vi "prepAO_imgtest.vi"() -> (0 "size(s)":i32[](array[numeric]))   [LabVIEW 2013]
uses:
  <vilib>/DAQmx/write.llb/DAQmx Write (Analog 2D DBL NChan NSamp).vi
  <vilib>/DAQmx/write.llb/DAQmx Write (Analog 1D DBL 1Chan NSamp).vi
  <vilib>/DAQmx/create/channels.llb/DAQmx Create Channel (AO-Voltage-Basic).vi
  <vilib>/DAQmx/configure/timing.llb/DAQmx Timing (Sample Clock).vi
  <vilib>/DAQmx/miscellaneous.llb/DAQmx Fill In Error Info.vi
  <resource>/objmgr/daqmx.rc
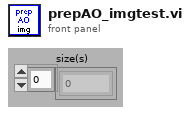
[diagram p1: front panel]
types:
  T1 = cluster{"Min Voltage sq (mV)":dbl, "Max voltage sq (mV)":dbl, "Duty cycle sq(%)":dbl, "Voltage freq. sq(Hz)":dbl, "# cycles sq":u32, "meastype":enum16{"sealtest hekcells", "sealtest neurons", "Manual", "from file"}, "sample rate":dbl, "amp":dbl, "sample mode":i32, "refreshbuffer":i32, "timeout":sgl, "patch":bool, "laserAO":bool, "shutter":bool, "488":bool, "532":bool, "640":bool, "Min Voltage tri (mV)":dbl, "Max voltage tri (mV)":dbl, "Voltage freq. tri(Hz)":dbl, "# cycles tri":u32, "Voltage step ":bool, "Voltage triangle":bool, "file":bool, "refreshrate":dbl, "sAOXY":dbl, "avpp":i32}
  T2 = cluster{"CH1 AI":tag, "CH1 CI":tag, "CH2 AI":tag, "CH2 CI":tag, "AI X":tag, "AI Y":tag, "AO X-Y":tag, "CH1ST":bool, "CH2ST":bool, "Sigcase":i16, "StageS":i32, "StageL":i32, "data dir":path, "Vp":tag, "Ip":tag, "AO CWlaser":tag, "AO VtoP":tag, "shutter":tag, "LT marker":tag, "488":tag, "532":tag, "640":tag}
  T3 = cluster{"Xpixels":i32, "Vx-min ref":dbl, "Vx-max ref":dbl, "P":dbl, "Ypixels":i32, "Vy-min ref":dbl, "Vy-max ref":dbl, "srate":dbl, "sAOxy":i32, "timeout":dbl, "type":string, "date":string, "time":string, "Colormap":u16, "Drawing Mode":u16, "Scanning Mode":u16, "square pixels":bool, "square matrix":bool, "Xpixels Img":i32, "Vx-min Img":dbl, "VX-max Img":dbl, "Ypixels Img":i32, "Vy-min Img":dbl, "Vy-max Img ":dbl, "Angle Img":dbl, "autoshutter":bool, "finite":bool, "cont":bool, "wavdet":bool, "measpoints":i32, "avpp":i32, "bufferAO":i32, "bufferAI":i32, "CH1":bool, "CH2":bool, "X":bool, "Y":bool, "Ip":bool, "Vp":bool, "starttick":u32, "waveform":path, "Vx-ref":dbl, "Vy-ref":dbl, "refreshrate":dbl, "refreshbuffer":i32, "tt_cycles":i32, "motorref":refnum<k7>, "mirrorswitch":refnum<k7>, "sample mode":i32, "maxbufferAI":i32, "sampletreshold":dbl}
  T4 = cluster{"VtoP":sgl[], "CWlasers":sgl[], "shutter":sgl[], "488":sgl[], "532":sgl[], "640":sgl[], "LT Marker":digitaldata}
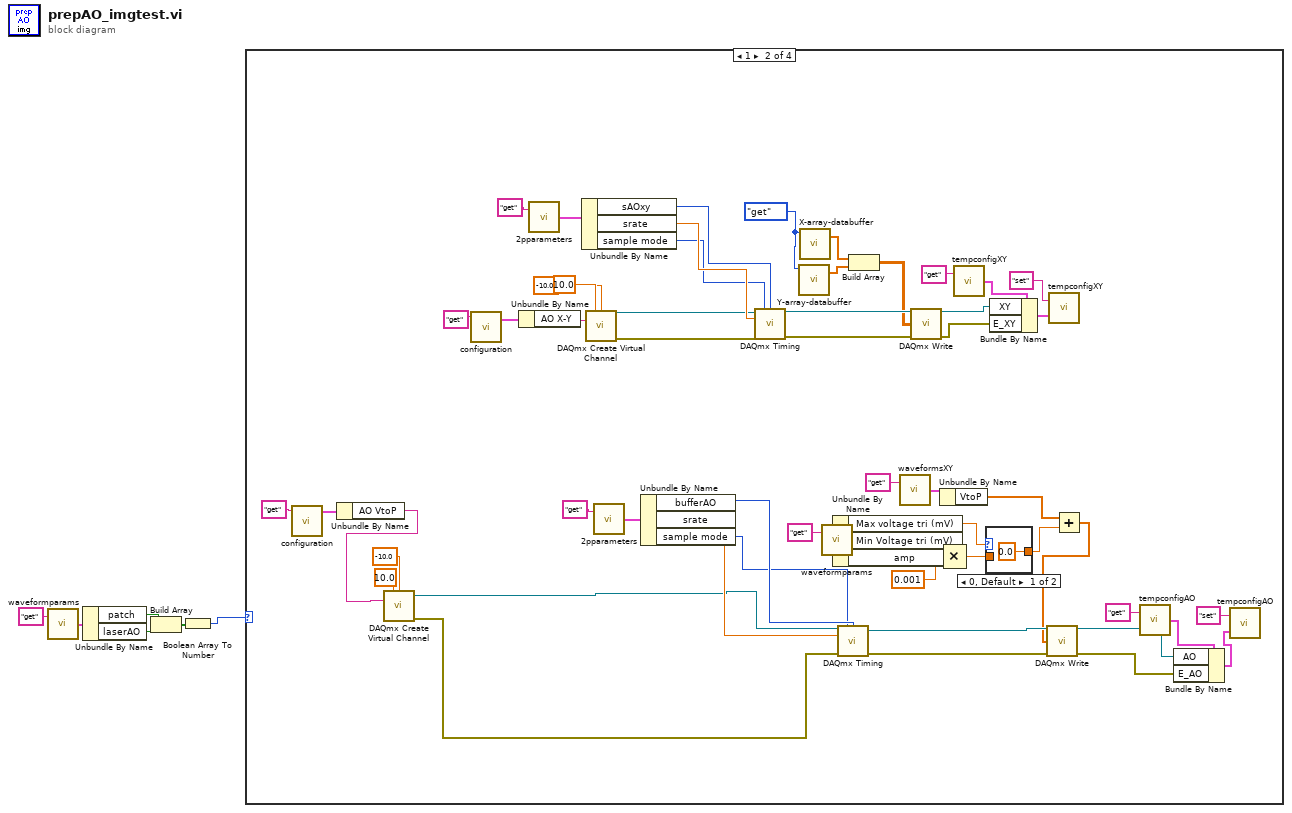
[diagram p0: block diagram]
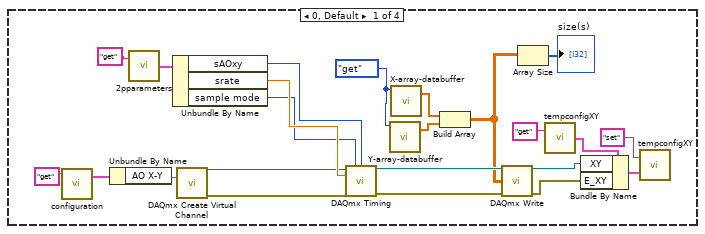
[diagram p2: hidden frame]
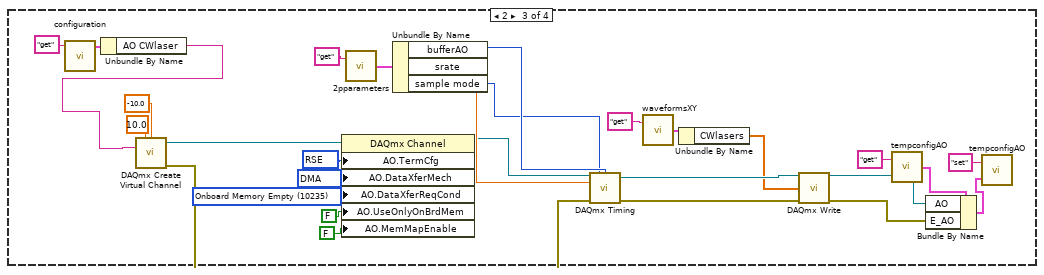
[diagram p4: hidden frame]
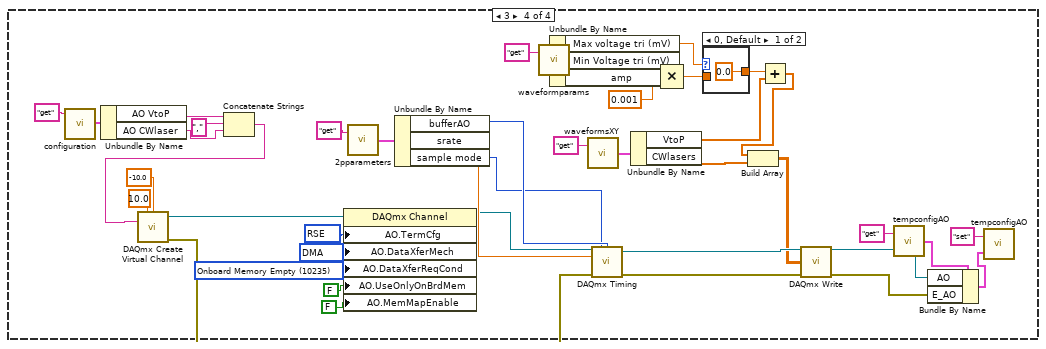
[diagram p5: hidden frame]
diagram:
  n1 = call "waveformparams.vi"("command"="get") -> ("Params out"=w4:T1)  [unwired: 1 in]
  n2 = Unbundle By Name(w4) -> ("patch"=w3:bool, "laserAO"=w2:bool)
  n3 = Build Array(w3, w2) -> (w1:bool[])
  n4 = Boolean Array To Number(Boolean array=w1) -> (number=w6:u32)
  n5 = case shown="1" w6 {
    frame 0, Default {
      w15 = enum16{"get", "set", "clear", "append"}."get" ("command")
      n6 = call "configuration.vi"("command"="get") -> ("config out"=w17:T2)  [unwired: 2 in, 1 out]
      n7 = Unbundle By Name(w17) -> ("AO X-Y"=w19:tag)
      n8 = call "2pparameters.vi"("command"="get") -> ("Params out"=w21:T3)  [unwired: 1 in]
      n9 = Unbundle By Name(w21) -> ("sAOxy"=w22:i32, "srate"=w29:dbl, "sample mode"=w9:i32)
      n10 = call-poly <vilib>:"DAQmx Create Virtual Channel.vi"("physical channels"=w19) -> ("task out"=w13:refnum<k21>, "error out"=w12:errorcluster)  [unwired: 13 in]
      n11 = call-poly <vilib>:"DAQmx Timing.vi"("task/channels in"=w13, "sample mode"=w9, "samples per channel"=w22, "rate"=w29, "error in"=w12) -> ("task out"=w11:refnum<k21>, "error out"=w10:errorcluster)  [unwired: 9 in]
      n12 = call "Y-array-databuffer.vi"("command"=w15) -> ("array out"=w16:dbl[])  [unwired: 3 in, 1 out]
      n13 = call "X-array-databuffer.vi"("command"=w15) -> ("array out"=w14:dbl[])  [unwired: 3 in, 1 out]
      n14 = Build Array(w14, w16) -> (w8:dbl[][])
      n15 = call-poly <vilib>:"DAQmx Write.vi"("task/channels in"=w11, "data"=w8, "error in"=w10) -> ("task out"=w24:refnum<k21>, "error out"=w23:errorcluster)  [unwired: 10 in, 1 out]
      n16 = Array Size(array=w8) -> (size(s)=→"size(s)":i32[])
      n17 = call "tempconfigXY.vi"("command"="get") -> ("Temp Config out"=w26:cluster{" XY":refnum<k21>, "E_XY":errorcluster})  [unwired: 1 in]
      n18 = Bundle By Name(cluster=w26, "XY"=w24, "E_XY"=w23) -> (w27:cluster{" XY":refnum<k21>, "E_XY":errorcluster})
      n19 = call "tempconfigXY.vi"("Temp Config in"=w27, "command"="set") -> ()  [unwired: 1 out]
    }
    frame 1 {
      w39 = enum16{"get", "set", "clear", "append"}."get" ("command")
      n20 = call "configuration.vi"("command"="get") -> ("config out"=w67:T2)  [unwired: 2 in, 1 out]
      n21 = Unbundle By Name(w67) -> ("AO VtoP"=w65:tag)
      n22 = call-poly <vilib>:"DAQmx Create Virtual Channel.vi"("maximum value"=10.0, "minimum value"=-10.0, "physical channels"=w65) -> ("task out"=w54:refnum<k21>, "error out"=w81:errorcluster)  [unwired: 6 in, 5 out]
      n23 = call "configuration.vi"("command"="get") -> ("config out"=w41:T2)  [unwired: 2 in, 1 out]
      n24 = Unbundle By Name(w41) -> ("AO X-Y"=w43:tag)
      n25 = call "2pparameters.vi"("command"="get") -> ("Params out"=w45:T3)  [unwired: 1 in]
      n26 = Unbundle By Name(w45) -> ("sAOxy"=w46:i32, "srate"=w53:dbl, "sample mode"=w32:i32)
      n27 = call-poly <vilib>:"DAQmx Create Virtual Channel.vi"("maximum value"=10.0, "minimum value"=-10.0, "physical channels"=w43) -> ("task out"=w37:refnum<k21>, "error out"=w36:errorcluster)  [unwired: 11 in]
      n28 = call "2pparameters.vi"("command"="get") -> ("Params out"=w74:T3)  [unwired: 1 in]
      n29 = Unbundle By Name(w74) -> ("bufferAO"=w76:i32, "srate"=w85:dbl, "sample mode"=w70:i32)
      n30 = call-poly <vilib>:"DAQmx Timing.vi"("task/channels in"=w37, "sample mode"=w32, "samples per channel"=w46, "rate"=w53, "error in"=w36) -> ("task out"=w35:refnum<k21>, "error out"=w33:errorcluster)  [unwired: 9 in]
      n31 = call "Y-array-databuffer.vi"("command"=w39) -> ("array out"=w40:dbl[])  [unwired: 3 in, 1 out]
      n32 = call "X-array-databuffer.vi"("command"=w39) -> ("array out"=w38:dbl[])  [unwired: 3 in, 1 out]
      n33 = call "waveformparams.vi"("command"="get") -> ("Params out"=w63:T1)  [unwired: 1 in]
      n34 = Unbundle By Name(w63) -> ("Max voltage tri (mV)"=w59:dbl, "Min Voltage tri (mV)"=w61:dbl, "amp"=w58:dbl)
      n35 = call-poly <vilib>:"DAQmx Timing.vi"("task/channels in"=w54, "sample mode"=w70, "samples per channel"=w76, "rate"=w85, "error in"=w81) -> ("task out"=w73:refnum<k21>, "error out"=w82:errorcluster)  [unwired: 2 in, 7 out]
      n36 = Build Array(w38, w40) -> (w34:dbl[][])
      n37 = call "waveformsXY.vi"("command"="get") -> ("waveforms out"=w69:T4)  [unwired: 1 in]
      n38 = call-poly <vilib>:"DAQmx Write.vi"("task/channels in"=w35, "data"=w34, "error in"=w33) -> ("task out"=w48:refnum<k21>, "error out"=w47:errorcluster)  [unwired: 10 in, 1 out]
      n39 = Unbundle By Name(w69) -> ("VtoP"=w57:sgl[])
      n40 = Compound Arithmetic op=MULTIPLY(w61, w58, 0.001 ("y")) -> (w60:dbl)
      n41 = call "tempconfigXY.vi"("command"="get") -> ("Temp Config out"=w50:cluster{" XY":refnum<k21>, "E_XY":errorcluster})  [unwired: 1 in]
      n42 = case shown="0, Default" w59 {
        tunnel: w60 -> [_ w87]
        tunnel: [0.0 w87] -> w56
        frame 0, Default {
        }
        frame 1 {
        }
      }
      n43 = Bundle By Name(cluster=w50, "XY"=w48, "E_XY"=w47) -> (w51:cluster{" XY":refnum<k21>, "E_XY":errorcluster})
      n44 = call "tempconfigXY.vi"("Temp Config in"=w51, "command"="set") -> ()  [unwired: 1 out]
      n45 = Add(x=w57, y=w56) -> (x+y=w55:dbl[])
      n46 = call-poly <vilib>:"DAQmx Write.vi"("task/channels in"=w73, "data"=w55, "error in"=w82) -> ("task out"=w84:refnum<k21>, "error out"=w83:errorcluster)  [unwired: 10 in, 1 out]
      n47 = call "tempconfigAO.vi"("command"="get") -> ("Temp Config out"=w79:cluster{"AO":refnum<k21>, "E_AO":errorcluster})  [unwired: 1 in]
      n48 = Bundle By Name(cluster=w79, "AO"=w84, "E_AO"=w83) -> (w80:cluster{"AO":refnum<k21>, "E_AO":errorcluster})
      n49 = call "tempconfigAO.vi"("Temp Config in"=w80, "command"="set") -> ()  [unwired: 1 out]
    }
    frame 2 {
      w97 = 10235 items=["Onboard Memory Empty"=10235, "Onboard Memory Half Full or Less"=10239, "Onboard Memory Less than Full"=10242] ("AO.DataXferReqCond 2")
      w96 = 10054 items=["DMA"=10054, "Interrupts"=10204, "Programmed I/O"=10264, "USB Bulk"=12590] ("AO.DataXferMech 2")
      w95 = 10083 items=["RSE"=10083, "Differential"=10106, "Pseudodifferential"=12529] ("AO.TermCfg")
      n50 = call "configuration.vi"("command"="get") -> ("config out"=w90:T2)  [unwired: 2 in, 1 out]
      n51 = Unbundle By Name(w90) -> ("AO CWlaser"=w88:tag)
      n52 = call-poly <vilib>:"DAQmx Create Virtual Channel.vi"("maximum value"=10.0, "minimum value"=-10.0, "physical channels"=w88) -> ("task out"=w102:refnum<k21>, "error out"=w112:errorcluster)  [unwired: 6 in, 5 out]
      n53 = property class="DAQmx Channel"(reference=w102, "AO.TermCfg"=w95, "AO.DataXferMech"=w96, "AO.DataXferReqCond"=w97, "AO.UseOnlyOnBrdMem"=FALSE, "AO.MemMapEnable"=FALSE) -> (reference out=w103:refnum<k21>)  [unwired: 1 in, 1 out]
      n54 = call "2pparameters.vi"("command"="get") -> ("Params out"=w105:T3)  [unwired: 1 in]
      n55 = Unbundle By Name(w105) -> ("bufferAO"=w107:i32, "srate"=w116:dbl, "sample mode"=w94:i32)
      n56 = call-poly <vilib>:"DAQmx Timing.vi"("task/channels in"=w103, "sample mode"=w94, "samples per channel"=w107, "rate"=w116, "error in"=w112) -> ("task out"=w104:refnum<k21>, "error out"=w113:errorcluster)  [unwired: 2 in, 7 out]
      n57 = call "waveformsXY.vi"("command"="get") -> ("waveforms out"=w93:T4)  [unwired: 1 in]
      n58 = Unbundle By Name(w93) -> ("CWlasers"=w91:sgl[])
      n59 = call-poly <vilib>:"DAQmx Write.vi"("task/channels in"=w104, "data"=w91, "error in"=w113) -> ("task out"=w115:refnum<k21>, "error out"=w114:errorcluster)  [unwired: 10 in, 1 out]
      n60 = call "tempconfigAO.vi"("command"="get") -> ("Temp Config out"=w110:cluster{"AO":refnum<k21>, "E_AO":errorcluster})  [unwired: 1 in]
      n61 = Bundle By Name(cluster=w110, "AO"=w115, "E_AO"=w114) -> (w111:cluster{"AO":refnum<k21>, "E_AO":errorcluster})
      n62 = call "tempconfigAO.vi"("Temp Config in"=w111, "command"="set") -> ()  [unwired: 1 out]
    }
    frame 3 {
      w140 = 10235 items=["Onboard Memory Empty"=10235, "Onboard Memory Half Full or Less"=10239, "Onboard Memory Less than Full"=10242] ("AO.DataXferReqCond 2")
      w139 = 10054 items=["DMA"=10054, "Interrupts"=10204, "Programmed I/O"=10264, "USB Bulk"=12590] ("AO.DataXferMech 2")
      w138 = 10083 items=["RSE"=10083, "Differential"=10106, "Pseudodifferential"=12529] ("AO.TermCfg")
      n63 = call "configuration.vi"("command"="get") -> ("config out"=w131:T2)  [unwired: 2 in, 1 out]
      n64 = Unbundle By Name(w131) -> ("AO VtoP"=w129:tag, "AO CWlaser"=w128:tag)
      n65 = Concatenate Strings(w129, "," ("string"), w128) -> (w127:string)
      n66 = call-poly <vilib>:"DAQmx Create Virtual Channel.vi"("maximum value"=10.0, "minimum value"=-10.0, "physical channels"=w127) -> ("task out"=w145:refnum<k21>, "error out"=w155:errorcluster)  [unwired: 6 in, 5 out]
      n67 = property class="DAQmx Channel"(reference=w145, "AO.TermCfg"=w138, "AO.DataXferMech"=w139, "AO.DataXferReqCond"=w140, "AO.UseOnlyOnBrdMem"=FALSE, "AO.MemMapEnable"=FALSE) -> (reference out=w146:refnum<k21>)  [unwired: 1 in, 1 out]
      n68 = call "2pparameters.vi"("command"="get") -> ("Params out"=w148:T3)  [unwired: 1 in]
      n69 = Unbundle By Name(w148) -> ("bufferAO"=w150:i32, "srate"=w159:dbl, "sample mode"=w137:i32)
      n70 = call "waveformparams.vi"("command"="get") -> ("Params out"=w125:T1)  [unwired: 1 in]
      n71 = Unbundle By Name(w125) -> ("Max voltage tri (mV)"=w121:dbl, "Min Voltage tri (mV)"=w123:dbl, "amp"=w120:dbl)
      n72 = call "waveformsXY.vi"("command"="get") -> ("waveforms out"=w134:T4)  [unwired: 1 in]
      n73 = call-poly <vilib>:"DAQmx Timing.vi"("task/channels in"=w146, "sample mode"=w137, "samples per channel"=w150, "rate"=w159, "error in"=w155) -> ("task out"=w147:refnum<k21>, "error out"=w156:errorcluster)  [unwired: 2 in, 7 out]
      n74 = Unbundle By Name(w134) -> ("VtoP"=w118:sgl[], "CWlasers"=w135:sgl[])
      n75 = Compound Arithmetic op=MULTIPLY(w123, w120, 0.001 ("y")) -> (w122:dbl)
      n76 = case shown="0, Default" w121 {
        tunnel: w122 -> [_ w161]
        tunnel: [0.0 w161] -> w119
        frame 0, Default {
        }
        frame 1 {
        }
      }
      n77 = Add(x=w119, y=w118) -> (x+y=w117:dbl[])
      n78 = Build Array(w117, w135) -> (w136:dbl[][])
      n79 = call-poly <vilib>:"DAQmx Write.vi"("task/channels in"=w147, "data"=w136, "error in"=w156) -> ("task out"=w158:refnum<k21>, "error out"=w157:errorcluster)  [unwired: 10 in, 1 out]
      n80 = call "tempconfigAO.vi"("command"="get") -> ("Temp Config out"=w153:cluster{"AO":refnum<k21>, "E_AO":errorcluster})  [unwired: 1 in]
      n81 = Bundle By Name(cluster=w153, "AO"=w158, "E_AO"=w157) -> (w154:cluster{"AO":refnum<k21>, "E_AO":errorcluster})
      n82 = call "tempconfigAO.vi"("Temp Config in"=w154, "command"="set") -> ()  [unwired: 1 out]
    }
  }
